vi "MCSA Spectra.vi"   [LabVIEW 2016, in "NI_EP_Motor Monitoring.lvlib"]
doc: "Calculates the zoom fast Fourier Transform (FFT) spectra of the motor. You must manually select the polymorphic instance you want to use."
uses:
  <vilib>/addons/Electrical Power/Motor Monitoring/NI_EP_Motor Monitoring.lvlib
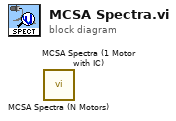
[diagram p0: block diagram]
diagram:
  n1 = call <vilib>:"MCSA Spectra (N Motors).vi"() -> ()  [unwired: 13 in, 3 out]
  n2 = call <vilib>:"MCSA Spectra (1 Motor with IC).vi"() -> ()  [unwired: 12 in, 4 out]
